vi "CI_Test.vi"() -> ()   [LabVIEW 2011]
uses:
  BeadTracker2.llb/GenericCameraConfigType.ctl
  BeadTracker2.llb/CIGrabParams.ctl
  qtrk/QTrk.llb/QTrkInstance.ctl
  BeadTracker2.llb/TrackingConfigType.ctl
  qtrk/QTrk.llb/QTrkLocalizationType.ctl
  qtrk/QTrk.llb/QTrkZCommandType.ctl
  qtrk/QTrk.llb/ResultManagerInstance.ctl
  BeadTracker2.llb/CmdData_NewFrame.ctl
  <vilib>/vision/Image Controls.llb/IMAQ Image.ctl
  BeadTracker2.llb/CmdEnum_CameraFrameType.ctl
  BeadTracker2.llb/CIGrabControlMsg.ctl
  BeadTracker2.llb/CIGrabControlMsgEnum.ctl
panel:
  in  "TrackingParameters":T1={"Corner-based bead pos (out)"=[], "QTrk Instance"={"QTrk Pointer"=0}, "Tracking Config"={"Number of steps"=0, "ZLUT stepsize (um)"=0.0, "Z correction factor"=0.0, "Start piezo Z (um)"=0.0, "Pixel size (nm)"=0.0, "2D Localization Type"=enum."Quadrant Interpolation", "Z Command (None)"=enum."Nothing"}, "ResultManager"={"InstancePtr"=0}, "Send to queue?"=TRUE}
  out "Frame #":i32
  out "Image":T7(plugin-control)
  in  "Display image?":bool=TRUE
  in  "Hardware ROI Index":i32
  in  "Corner-based bead pos (out)":cluster{"X":i32, "Y":i32}[](array[cluster])
  in  "GenericCameraConfig":T8={"Framerate (Hz)"=60, "Exposure time (us)"=10000, "Image size"={"Width"=1280, "Height"=1024}}
  in  "Config":bool
  out "Camera state":variant
  in  "Close":bool
  in  "Grab":bool
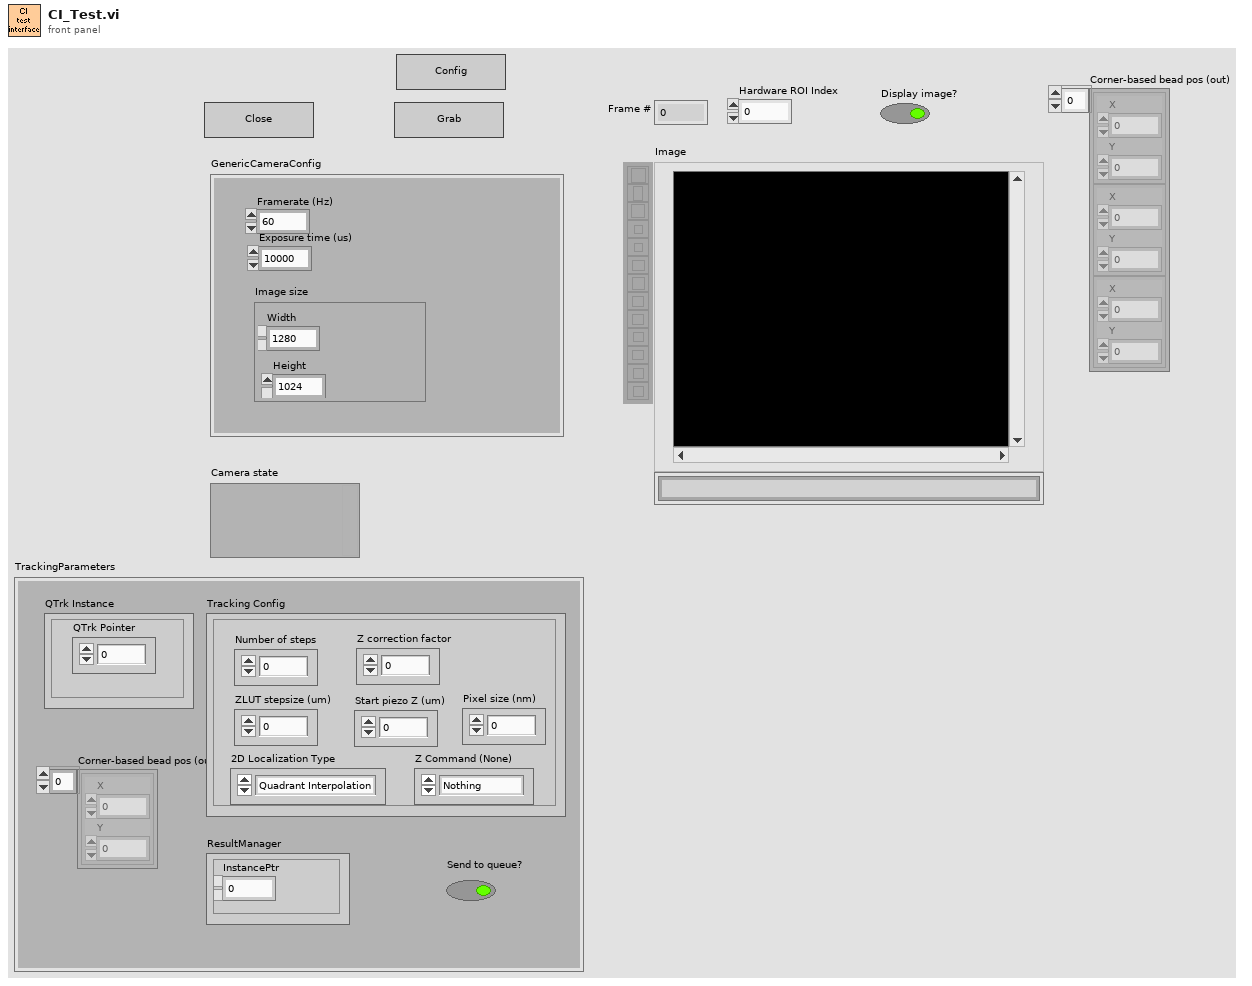
[diagram p1: front panel]
types:
  T1 = typedef "CIGrabParams.ctl" = cluster{"Corner-based bead pos (out)":cluster{"X":i32, "Y":i32}[], "QTrk Instance":T2, "Tracking Config":T3, "ResultManager":T6, "Send to queue?":bool}
  T2 = typedef "QTrkInstance.ctl" = cluster{"QTrk Pointer":u64}
  T3 = typedef "TrackingConfigType.ctl" = cluster{"Number of steps":i32, "ZLUT stepsize (um)":sgl, "Z correction factor":sgl, "Start piezo Z (um)":sgl, "Pixel size (nm)":sgl, "2D Localization Type":T4, "Z Command (None)":T5}
  T4 = typedef "QTrkLocalizationType.ctl" = enum16{"Center-of-Mass", "1D Cross-Correlation", "Quadrant Interpolation", "Gaussian 2D MLE"}
  T5 = typedef "QTrkZCommandType.ctl" = enum16{"Nothing", "ComputeZ", "BuildZLUT"}
  T6 = typedef "ResultManagerInstance.ctl" = cluster{"InstancePtr":u64}
  T7 = typedef "IMAQ Image.ctl" = refnum<image>
  T8 = typedef "GenericCameraConfigType.ctl" = cluster{"Framerate (Hz)":i32, "Exposure time (us)":i32, "Image size":cluster{"Width":i32, "Height":i32}}
  T9 = typedef "CmdData_NewFrame.ctl" = cluster{"Buffer Image":T7, "Frame #":i32, "Hardware ROI Index":i32, "Timestamp":dbl, "Type":T10}
  T10 = typedef "CmdEnum_CameraFrameType.ctl" = enum16{"Full", "HardwareROI", "EndGrabMarker"}
  T11 = typedef "CIGrabControlMsg.ctl" = cluster{"Msg":T12}
  T12 = typedef "CIGrabControlMsgEnum.ctl" = enum16{"Stop", "EnableTracking", "DisableTracking"}
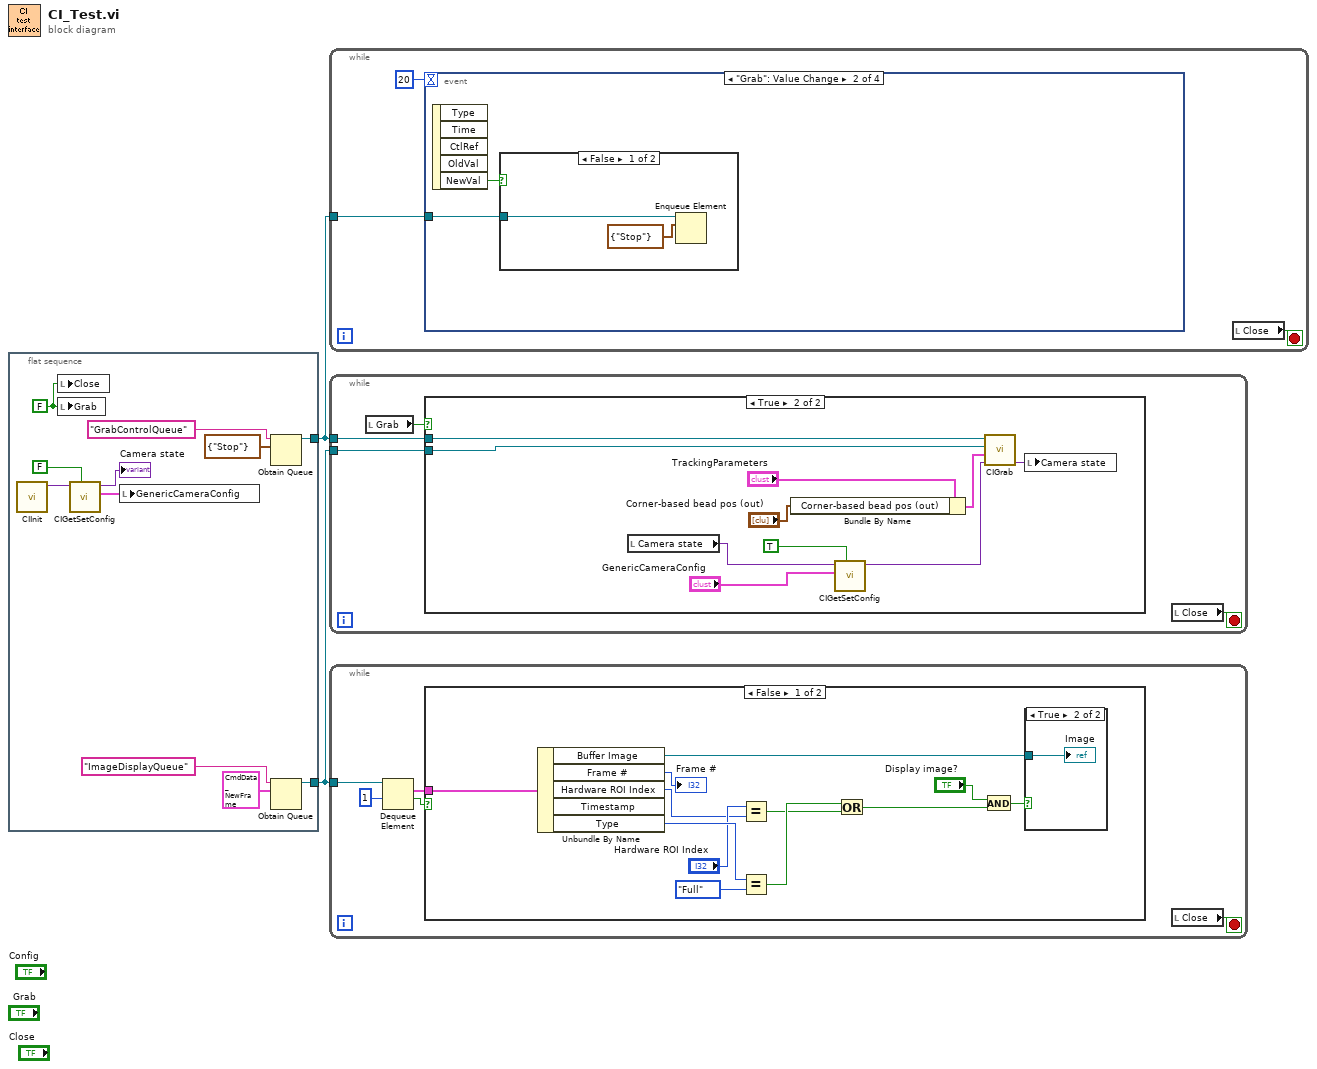
[diagram p0: block diagram]
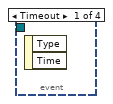
[diagram p5: hidden frame]
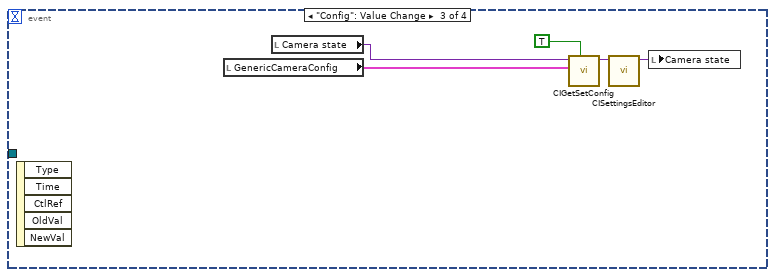
[diagram p7: hidden frame]
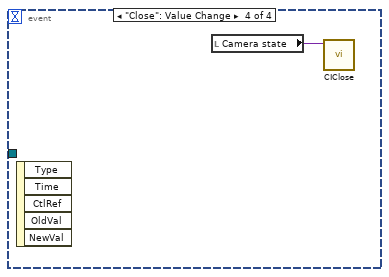
[diagram p8: hidden frame]
diagram:
  n1 = flat-sequence {
    tunnel: [w11] -> w1
    tunnel: [w8] -> w2
    frame #0 {
      w7 = FALSE ("Close")
      n2 = call "CIInit.vi"() -> ("Camera data (out)"=w6:variant)  [unwired: 11 in]
      n3 = local write "Close"(w7) -> ()
      n4 = local write "Grab"(w7) -> ()
      n5 = call "CIGetSetConfig.vi"("Set? (F)"=FALSE ("Set?"), "Camera state"=w6) -> ("GenericCameraConfig (out)"=w3:T8, "Camera state (out)"=→"Camera state":variant)  [unwired: 8 in]
      n6 = local write "GenericCameraConfig"(w3) -> ()
      n7 = Obtain Queue(name (unnamed)="GrabControlQueue", element data type=T11 {"Msg"=enum."Stop"} ("GrabControlMsg")) -> (queue out=w11:refnum<queue>)  [unwired: 3 in, 2 out]
      n8 = Obtain Queue(name (unnamed)="ImageDisplayQueue", element data type=T9 {"Buffer Image"=refnum, "Frame #"=0, "Hardware ROI Index"=0, "Timestamp"=0.0, "Type"=enum."Full"} ("Cluster")) -> (queue out=w8:refnum<queue>)  [unwired: 3 in, 2 out]
    }
  }
  n9 = while {
    tunnel: w1 -> [w14]
    stop <- w15 stop-if-true
    n10 = event shown="[1] \"Grab\": Value Change" {
      selector: _ -> [_ _ _ _]
      dyn-events: _ -> [_ _ _ _]
      timeout: 20 -> [_ _ _ _]
      tunnel: w14 -> [_ w17 _ _]
      event Timeout {
        n11 = event-data() -> ()  [unwired: 1 in, 2 out]
      }
      event "Grab": Value Change {
        n12 = event-data() -> ("NewVal"=w18:bool)  [unwired: 1 in, 4 out]
        n13 = case shown="False" w18 {
          tunnel: w17 -> [w20 _]
          frame False {
            n14 = Enqueue Element(queue=w20, element=T11 {"Msg"=enum."Stop"}) -> ()  [unwired: 2 in, 3 out]
          }
          frame True {
          }
        }
      }
      event "Config": Value Change {
        n15 = event-data() -> ()  [unwired: 1 in, 5 out]
        n16 = local read "GenericCameraConfig"() -> (w23:T8)
        n17 = local read "Camera state"() -> (w24:variant)
        n18 = call "CIGetSetConfig.vi"("Set? (F)"=TRUE ("Set?"), "GenericCameraConfig"=w23, "Camera state"=w24) -> ("Camera state (out)"=w21:variant)  [unwired: 7 in, 1 out]
        n19 = call "CISettingsEditor.vi"("Camera state"=w21) -> ("Camera state (out)"=w25:variant)  [unwired: 10 in]
        n20 = local write "Camera state"(w25) -> ()
      }
      event "Close": Value Change {
        n21 = event-data() -> ()  [unwired: 1 in, 5 out]
        n22 = local read "Camera state"() -> (w26:variant)
        n23 = call "CIClose.vi"("Camera data"=w26) -> ()  [unwired: 11 in]
      }
    }
    n24 = local read "Close"() -> (w15:bool)
  }
  n25 = while {
    tunnel: w1 -> [w29]
    tunnel: w2 -> [w28]
    stop <- w27 stop-if-true
    n26 = local read "Grab"() -> (w30:bool)
    n27 = case shown="True" w30 {
      tunnel: w29 -> [_ w40]
      tunnel: w28 -> [_ w39]
      frame False {
      }
      frame True {
        n28 = local read "Camera state"() -> (w35:variant)
        n29 = Bundle By Name(cluster="TrackingParameters", "Corner-based bead pos (out)"="Corner-based bead pos (out)") -> (w36:T1)
        n30 = call "CIGetSetConfig.vi"("Set? (F)"=TRUE, "GenericCameraConfig"="GenericCameraConfig", "Camera state"=w35) -> ("Camera state (out)"=w32:variant)  [unwired: 7 in, 1 out]
        n31 = call "CIGrab.vi"("Camera data"=w32, "TrackingParameters"=w36, "Output Queue"=w39, "GrabControlQueue"=w40) -> ("Camera (out)"=w31:variant)  [unwired: 7 in]
        n32 = local write "Camera state"(w31) -> ()
      }
    }
    n33 = local read "Close"() -> (w27:bool)
  }
  n34 = while {
    tunnel: w2 -> [w44]
    stop <- w45 stop-if-true
    n35 = Dequeue Element(queue=w44, timeout in ms (-1)=1) -> (element=w41:T9, timed out?=w42:bool)  [unwired: 1 in, 2 out]
    n36 = case shown="False" w42 {
      tunnel: w41 -> [w57 _]
      frame False {
        n37 = Unbundle By Name(w57) -> ("Buffer Image"=w46:T7, "Frame #"=→"Frame #":i32, "Hardware ROI Index"=w51:i32, "Type"=w55:T10)  [unwired: 1 out]
        n38 = Equal?(x="Hardware ROI Index", y=w51) -> (x = y?=w50:bool)
        n39 = Equal?(x=w55, y=CmdEnum_CameraFrameType."Full") -> (x = y?=w53:bool)
        n40 = Or(x=w53, y=w50) -> (x .or. y?=w48:bool)
        n41 = And(x="Display image?", y=w48) -> (x .and. y?=w47:bool)
        n42 = case shown="True" w47 {
          tunnel: w46 -> [_ w58]
          frame False {
          }
          frame True {
            "Image" <- w58
          }
        }
      }
      frame True {
      }
    }
    n43 = local read "Close"() -> (w45:bool)
  }
